vi "读配置.vi"(8 "error in":errorcluster) -> (0 "error out":errorcluster, 1 "ADC_GAIN":u32, 2 "LDO_TRIM":u32, 3 "return":i32)   [LabVIEW 2016]
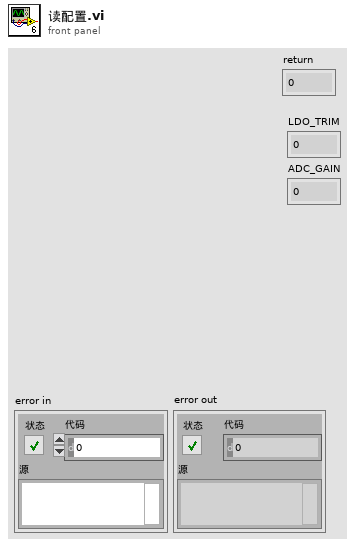
[diagram p1: front panel]
types:
  T1 = cluster{"byCmdType":u8, "bySubCmd":u8, "byPara":u8, "byAddr_h":u8, "byAddr_l":u8, "byAddr_ll":u8, "byLen_h":u8, "byLen_l":u8}
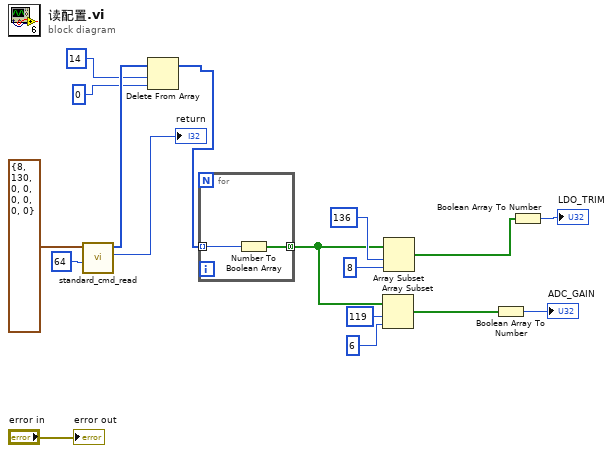
[diagram p0: block diagram]
diagram:
  n1 = call "standard_cmd_read.vi"("dwLen"=u32 64, "cmd_std_header_t"=T1 {"byCmdType"=8, "bySubCmd"=130, "byPara"=0, "byAddr_h"=0, "byAddr_l"=0, "byAddr_ll"=0, "byLen_h"=0, "byLen_l"=0}) -> ("return"=→"return":i32, "data out"=w4:u8[])  [unwired: 7 in, 1 out]
  n2 = Delete From Array(array=w4, length=14, index=0) -> (array with subset deleted=w1:u8[])  [unwired: 1 out]
  n3 = for {
    tunnel: w1 -> [w19] mode=indexing
    tunnel: [w18] -> w12 mode=concatenating
    n4 = Number To Boolean Array(number=w19) -> (Boolean array=w18:bool[])
  }
  n5 = Array Subset(array=w12, index=119, length=6) -> (w5:bool[])
  n6 = Array Subset(array=w12, index=136, length=8) -> (w6:bool[])
  n7 = Boolean Array To Number(Boolean array=w5) -> (number=→"ADC_GAIN":u32)
  n8 = Boolean Array To Number(Boolean array=w6) -> (number=→"LDO_TRIM":u32)
  "error out" <- "error in"
